vi "tests.TimeoutTimer.vi"() -> ()   [LabVIEW 2017]
panel:
  out "time esliped?":dbl
  in  "timeout(s)":dbl=5.0
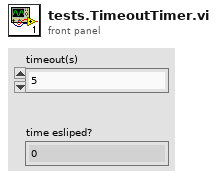
[diagram p1: front panel]
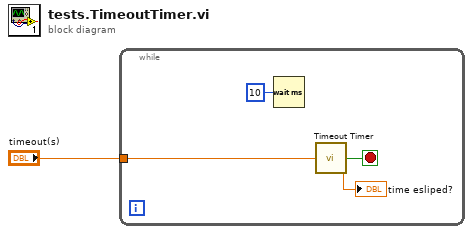
[diagram p0: block diagram]
diagram:
  n1 = while {
    tunnel: "timeout(s)" -> [w5]
    stop <- w4 stop-if-true
    n2 = Wait (ms)(milliseconds to wait=u32 10) -> ()  [unwired: 1 out]
    n3 = call "Timeout Timer.vi"("timeout(s)"=w5) -> ("timeout?"=w4:bool, "time esliped?"=→"time esliped?":dbl)  [unwired: 7 in]
  }
